vi "Result_Test.vi"(8 "error in (no error)":errorcluster caption="entrée d'erreur (pas d'erreur)", 11 "Get_Voltage en entrée":refnum<class "P2056_Wait_Start.lvclass">) -> (0 "error out":errorcluster caption="sortie d'erreur", 3 "Get_Voltage en sortie":refnum<class "P2056_Wait_Start.lvclass">)   [LabVIEW 2020, in "Library Test.lvlib" / "P2056_Wait_Start.lvclass"]
uses:
  P2056_Wait_Start.lvclass
  C:/Users/ngarcin/OneDrive - Altyor/Standard TB/Class/Test/Test (Default)/Test (Default).lvclass
  P2056_Send_Command_UART/P2056_Send_Command_UART.lvclass
  P2056_Wait_Start.lvclass/P2056_Wait_Start.ctl
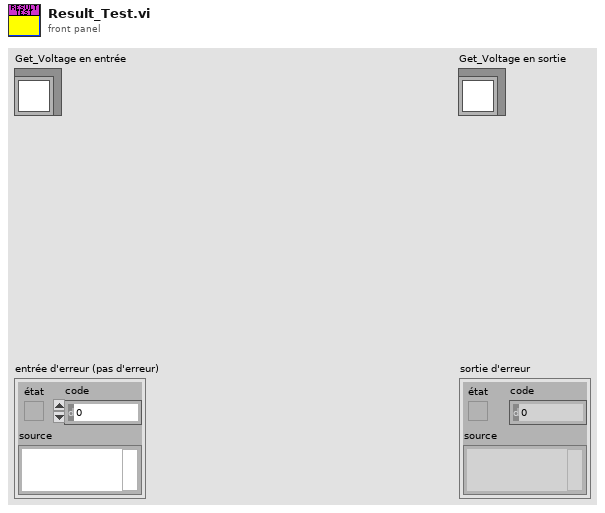
[diagram p1: front panel]
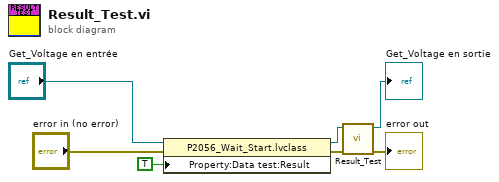
[diagram p0: block diagram]
diagram:
  n1 = property class="P2056_Wait_Start.lvclass"(reference="Get_Voltage en entrée", error in="error in (no error)", "Property:Data test:Result"=TRUE ("Result")) -> (reference out=w5:refnum<class "P2056_Wait_Start.lvclass">, error out=w6:errorcluster)
  n2 = call-parent "Result_Test.vi"("error in (no error)"=w6, "Get_Voltage en entrée"=w5) -> ("error out"=→"error out":errorcluster, "Get_Voltage en sortie"=→"Get_Voltage en sortie":refnum<class "P2056_Wait_Start.lvclass">)  [unwired: 8 in]
